vi "UpdateListNames.vi"(8 "error in (no error)":errorcluster, 10 "Item Names":string[](array[string]), 11 "MC-ExternClient in":refnum<class "MC-ExternClient.lvclass">) -> (0 "error out":errorcluster, 3 "MC-ExternClient out":refnum<class "MC-ExternClient.lvclass">)   [LabVIEW 2020, in "MC-ExternClient.lvlib" / "MC-ExternClient.lvclass"]
uses:
  MC-ExternClient.lvclass
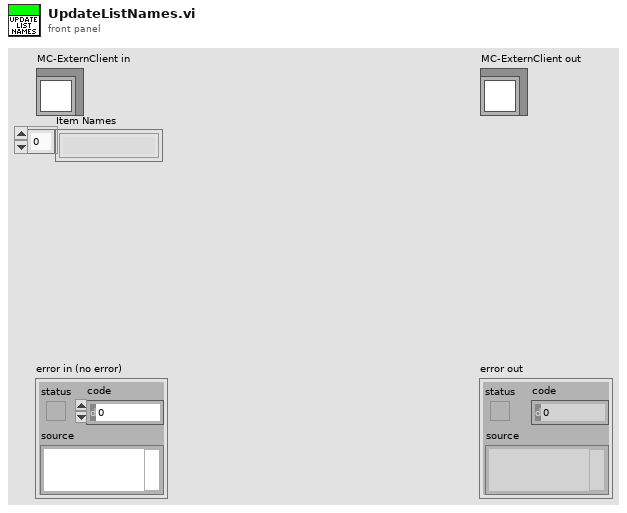
[diagram p1: front panel]
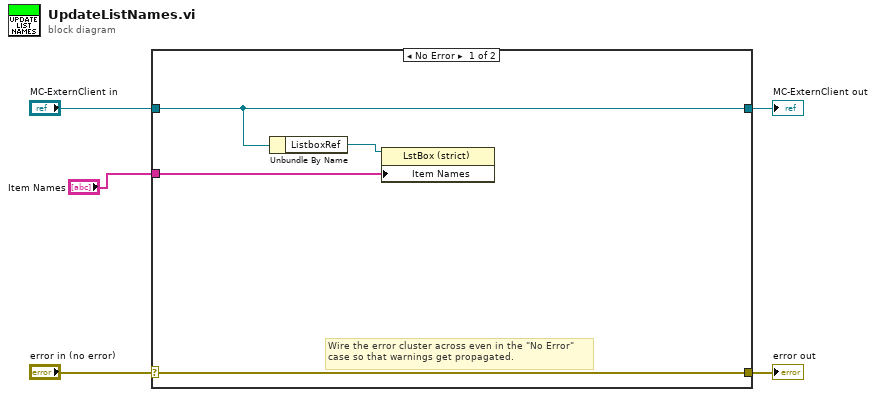
[diagram p0: block diagram]
diagram:
  n1 = case shown="No Error" "error in (no error)" {
    selector: "error in (no error)" -> [w9 w11]
    tunnel: [w9 w11] -> w4
    tunnel: [w8 w10] -> w2
    tunnel: "MC-ExternClient in" -> [w8 w10]
    tunnel: "Item Names" -> [w6 _]
    frame No Error {
      # "Wire the error cluster across even in the \"No Error\"\ncase so that warnings get propagated."
      n2 = Unbundle By Name(w8) -> ("ListboxRef"=w7:refnum<vi>)
      n3 = property class="LstBox (strict)"(reference=w7, "Item Names"=w6) -> ()  [unwired: 1 in, 2 out]
    }
    frame Error {
    }
  }
  "error out" <- w4
  "MC-ExternClient out" <- w2
